vi "FG Client Configurations.vi"(7 "action":T1, 8 "error in":errorcluster, 10 "mark configured? (T)":bool=TRUE, 11 "server ID":string) -> (0 "error out":errorcluster, 2 "group name":string, 3 "configured?":bool)   [LabVIEW 2010, in "NI_CCC.lvlib"]
uses:
  NI_CCC.lvlib
  FG Client Configurations Action.ctl
  Client Config Status.ctl
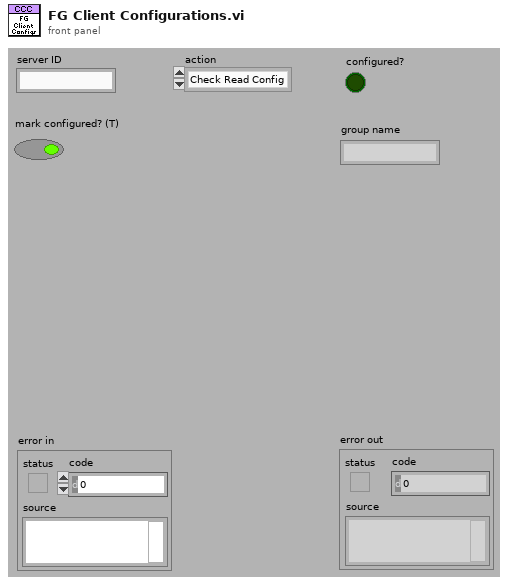
[diagram p1: front panel]
types:
  T1 = typedef "NI_CCC.lvlib/FG Client Configurations Action.ctl" = enum16{"Check Read Config", "Check Write Config", "Mark Read Config", "Mark Write Config"}
  T2 = typedef "NI_CCC.lvlib/Client Config Status.ctl" = cluster{"read configured":bool, "write configured":bool, "read group name":string, "write group name":string}
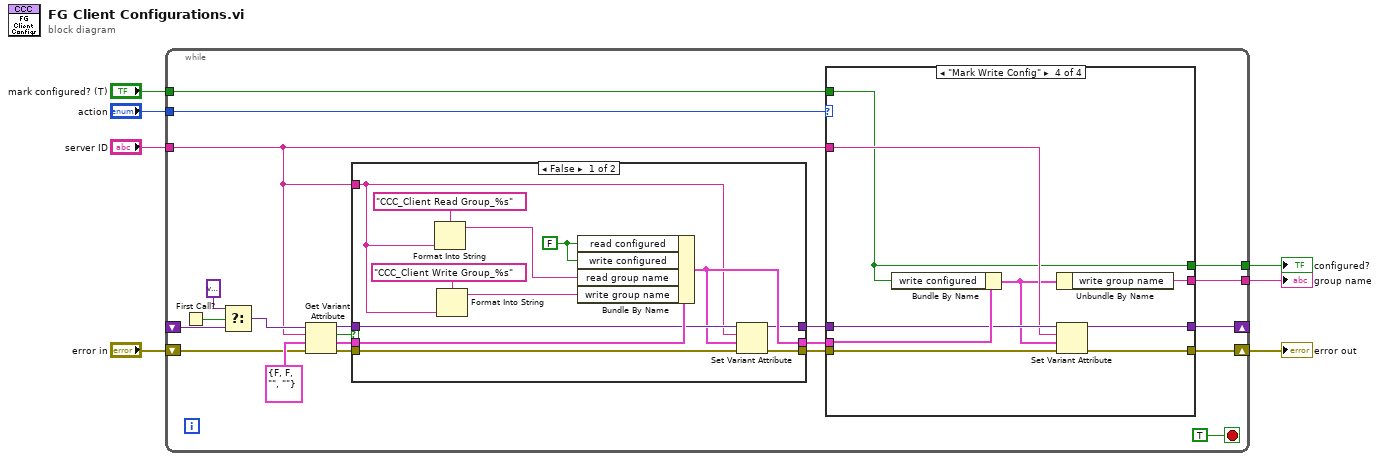
[diagram p0: block diagram]
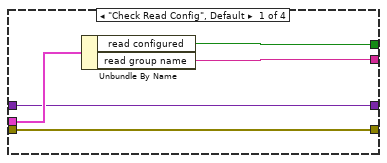
[diagram p3: hidden frame]
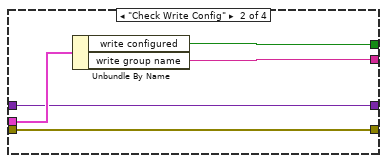
[diagram p4: hidden frame]
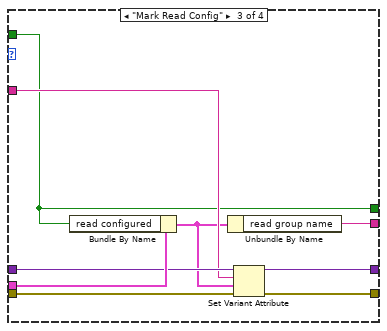
[diagram p5: hidden frame]
diagram:
  n1 = while {
    tunnel: "action" -> [w28]
    tunnel: "server ID" -> [w8]
    shift-right: [w10] -> w2
    shift-left: "error in" -> [w20]
    shift-right: [w24] -> _
    shift-left: _ -> [w23]
    tunnel: [w12] -> w3
    tunnel: [w11] -> w4
    tunnel: "mark configured? (T)" -> [w9]
    stop <- TRUE stop-if-true
    n2 = First Call?() -> (First Call?: T/F=w27:bool)
    n3 = Select(t=variant ("Variant"), s=w27, f=w23) -> (s? t:f=w21:variant)
    n4 = Get Variant Attribute(Variant=w21, name=w8, default value (empty Variant)=T2 {"read configured"=FALSE, "write configured"=FALSE, "read group name"="", "write group name"=""} ("status"), error in=w20) -> (duplicate Variant=w18:variant, found=w19:bool, value=w17:T2, error out=w16:errorcluster)
    n5 = case shown="False" w19 {
      tunnel: w18 -> [w34 w43]
      tunnel: w17 -> [w35 w41]
      tunnel: w16 -> [w32 w42]
      tunnel: [w30 w43] -> w15
      tunnel: [w31 w42] -> w14
      tunnel: [w33 w41] -> w13
      tunnel: w8 -> [w29 _]
      frame False {
        w36 = FALSE ("read configured")
        n6 = Format Into String(format string="CCC_Client Read Group_%s", w29) -> (resulting string=w38:string)  [unwired: 2 in, 1 out]
        n7 = Format Into String(format string="CCC_Client Write Group_%s", w29) -> (resulting string=w37:string)  [unwired: 2 in, 1 out]
        n8 = Bundle By Name(cluster=w35, "read configured"=w36, "write configured"=w36, "read group name"=w38, "write group name"=w37) -> (w33:T2)
        n9 = Set Variant Attribute(Variant=w34, name=w29, value=w33, error in=w32) -> (Variant out=w30:variant, error out=w31:errorcluster)  [unwired: 1 out]
      }
      frame True {
      }
    }
    n10 = case shown="\"Mark Write Config\"" w28 {
      tunnel: w8 -> [_ _ w57 w68]
      tunnel: [w45 w51 w58 w67] -> w24
      tunnel: w15 -> [w45 w51 w61 w69]
      tunnel: w14 -> [w44 w49 w60 w71]
      tunnel: w13 -> [w48 w53 w62 w70]
      tunnel: [w47 w52 w54 w63] -> w12
      tunnel: [w46 w50 w55 w64] -> w11
      tunnel: [w44 w49 w59 w66] -> w10
      tunnel: w9 -> [_ _ w54 w63]
      frame "Check Read Config", Default {
        n11 = Unbundle By Name(w48) -> ("read configured"=w47:bool, "read group name"=w46:string)
      }
      frame "Check Write Config" {
        n12 = Unbundle By Name(w53) -> ("write configured"=w52:bool, "write group name"=w50:string)
      }
      frame "Mark Read Config" {
        n13 = Bundle By Name(cluster=w62, "read configured"=w54) -> (w56:T2)
        n14 = Unbundle By Name(w56) -> ("read group name"=w55:string)
        n15 = Set Variant Attribute(Variant=w61, name=w57, value=w56, error in=w60) -> (Variant out=w58:variant, error out=w59:errorcluster)  [unwired: 1 out]
      }
      frame "Mark Write Config" {
        n16 = Bundle By Name(cluster=w70, "write configured"=w63) -> (w65:T2)
        n17 = Unbundle By Name(w65) -> ("write group name"=w64:string)
        n18 = Set Variant Attribute(Variant=w69, name=w68, value=w65, error in=w71) -> (Variant out=w67:variant, error out=w66:errorcluster)  [unwired: 1 out]
      }
    }
  }
  "error out" <- w2
  "configured?" <- w3
  "group name" <- w4
